vi "CNP LAB 4.vi"() -> ()   [LabVIEW 2023]
panel:
  in  "CNP":string
  out "Luna":bool
  out "Gen":string
  out "Nr cifre":bool
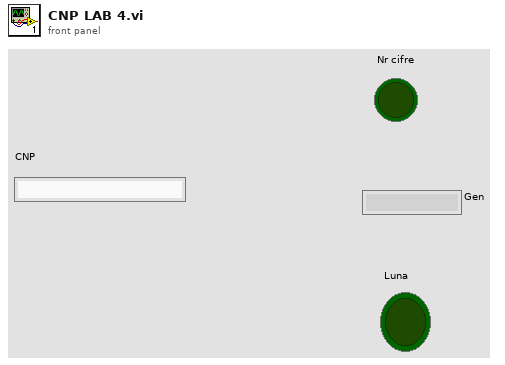
[diagram p1: front panel]
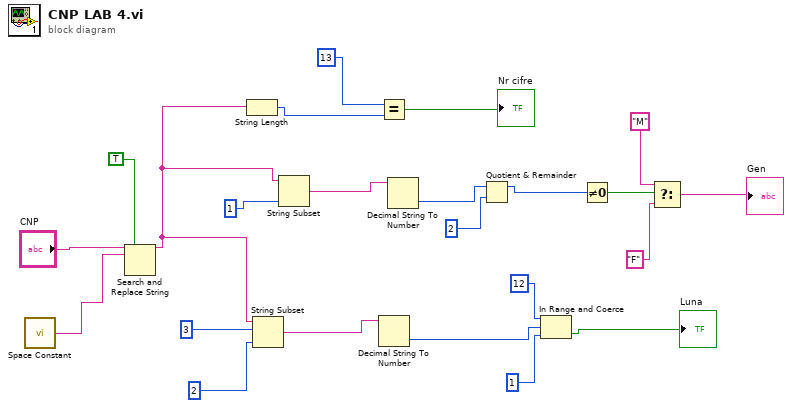
[diagram p0: block diagram]
diagram:
  n1 = call <vilib>:"Space Constant.vi"() -> ("String"=w1:string)
  n2 = Search and Replace String(replace all?=TRUE, input string="CNP", search string=w1) -> (result string=w10:string)  [unwired: 5 in, 3 out]
  n3 = String Length(string=w10) -> (length=w20:i32)
  n4 = String Subset(string=w10, offset (0)=3, length (rest)=2) -> (substring=w7:string)
  n5 = String Subset(string=w10, length (rest)=1) -> (substring=w17:string)  [unwired: 1 in]
  n6 = Equal?(x=13, y=w20) -> (x = y?=→"Nr cifre":bool)
  n7 = Decimal String To Number(string=w7) -> (number=w4:i32)  [unwired: 2 in, 1 out]
  n8 = Decimal String To Number(string=w17) -> (number=w2:i32)  [unwired: 2 in, 1 out]
  n9 = Quotient & Remainder(x=w2, y=2) -> (x-y*floor(x/y)=w15:i32)  [unwired: 1 out]
  n10 = In Range and Coerce(upper limit=12, x=w4, lower limit=1) -> (In Range?=→"Luna":bool)  [unwired: 1 out]
  n11 = Not Equal To 0?(x=w15) -> (x != 0?=w12:bool)
  n12 = Select(t="M", s=w12, f="F") -> (s? t:f=→"Gen":string)
